vi "RichToFlatnixnet_grpc_ReadStateRequest.vi"(5 "OutputClusterType":T1, 11 "InputCluster":T4) -> (3 "OutputCluster":T1)   [LabVIEW 2025, in "grpc-xnet_client.lvlib"]
uses:
  grpc-xnet_client.lvlib
  nixnet_grpc_ReadStateRequest.ctl
  nixnet_grpc_ReadStateRequest_state_id_enum/nixnet_grpc_ReadStateRequest_state_id_enum.lvclass
  nidevice_grpc_Session.ctl
  nixnet_grpc_ReadStateRequest_Flat.ctl
  nidevice_grpc_Session_Flat.ctl
  nixnet_grpc_ReadState.ctl
  nixnet_grpc_ReadStateRequest_state_id_enum/nixnet_grpc_ReadStateRequest_state_id_enum.lvclass/nixnet_grpc_ReadStateRequest_state_id_enum.ctl
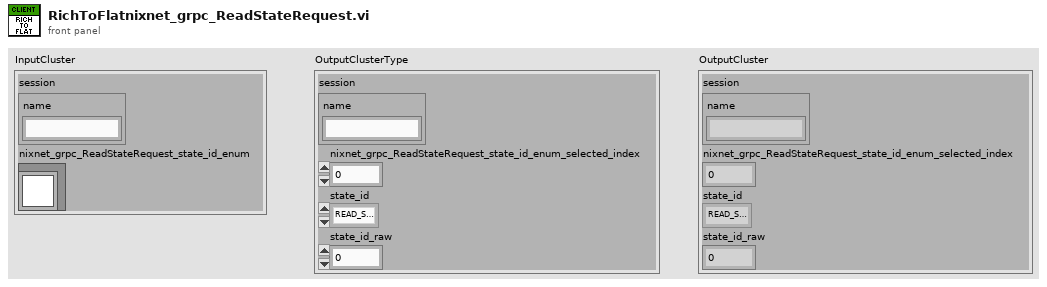
[diagram p1: front panel]
types:
  T1 = typedef "grpc-xnet_client.lvlib/nixnet_grpc_ReadStateRequest_Flat.ctl" = cluster{"session":T2, "nixnet_grpc_ReadStateRequest_state_id_enum_selected_index":i32, "state_id":T3, "state_id_raw":u32}
  T2 = typedef "grpc-xnet_client.lvlib/nidevice_grpc_Session_Flat.ctl" = cluster{"name":string}
  T3 = typedef "grpc-xnet_client.lvlib/nixnet_grpc_ReadState.ctl" = enum32{"READ_STATE_UNSPECIFIED", "READ_STATE_TIME_CURRENT", "READ_STATE_TIME_COMMUNICATING", "READ_STATE_TIME_START", "READ_STATE_SESSION_INFO", "READ_STATE_TIME_CURRENT_2", "READ_STATE_TIME_COMMUNICATING_2", "READ_STATE_TIME_START_2", "READ_STATE_CAN_COMM", "READ_STATE_FLEX_RAY_COMM", "READ_STATE_FLEX_RAY_STATS", "READ_STATE_LIN_COMM", "READ_STATE_J1939_COMM"}
  T4 = typedef "grpc-xnet_client.lvlib/nixnet_grpc_ReadStateRequest.ctl" = cluster{"session":T5, "nixnet_grpc_ReadStateRequest_state_id_enum":refnum<class "nixnet_grpc_ReadStateRequest_state_id_enum.lvclass">}
  T5 = typedef "grpc-xnet_client.lvlib/nidevice_grpc_Session.ctl" = cluster{"name":string}
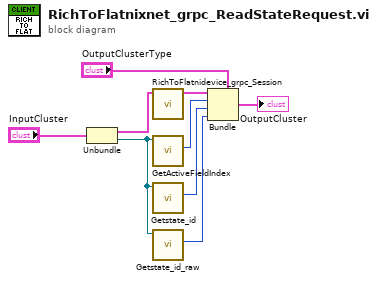
[diagram p0: block diagram]
diagram:
  n1 = Unbundle "Unbundle"("InputCluster") -> ("session"=w6:T5, "nixnet_grpc_ReadStateRequest_state_id_enum"=w4:refnum<class "nixnet_grpc_ReadStateRequest_state_id_enum.lvclass">)
  n2 = call "RichToFlatnidevice_grpc_Session.vi"("InputCluster"=w6) -> ("OutputCluster"=w5:T2)  [unwired: 10 in]
  n3 = call "GetActiveFieldIndex.vi"("OneOfTemplate in"=w4) -> ("Active Field Index"=w3:i32)  [unwired: 8 in, 2 out]
  n4 = call "Getstate_id.vi"("OneOfTemplate in"=w4) -> ("Get_Val"=w2:T3)  [unwired: 8 in, 2 out]
  n5 = call "Getstate_id_raw.vi"("OneOfTemplate in"=w4) -> ("Get_Val"=w1:u32)  [unwired: 8 in, 2 out]
  n6 = Bundle "Bundle"(cluster="OutputClusterType", "session"=w5, "nixnet_grpc_ReadStateRequest_state_id_enum_selected_index"=w3, "state_id"=w2, "state_id_raw"=w1) -> (→"OutputCluster":T1)
